vi "Unpack Goal Target Info.vi"(6 "Right Goal":T1, 8 "Left Goal":T1) -> (0 "Goal Found":bool, 1 "Target Y Angle (Cam relative)":dbl, 2 "Target X Angle (Cam relative)":dbl)   [LabVIEW 2013]
uses:
  Common Code/Goal Info.ctl
  Robot Global Data.vi
panel:
  # "CAMERA RELATIVE"
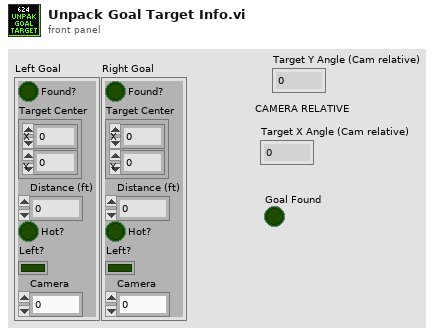
[diagram p1: front panel]
types:
  T1 = typedef "Goal Info.ctl" = cluster{"Found?":bool, "Target Center":cluster{"X":dbl, "Y":dbl}, "Distance (ft)":dbl, "Hot?":bool, "Left?":bool, "Camera":i16}
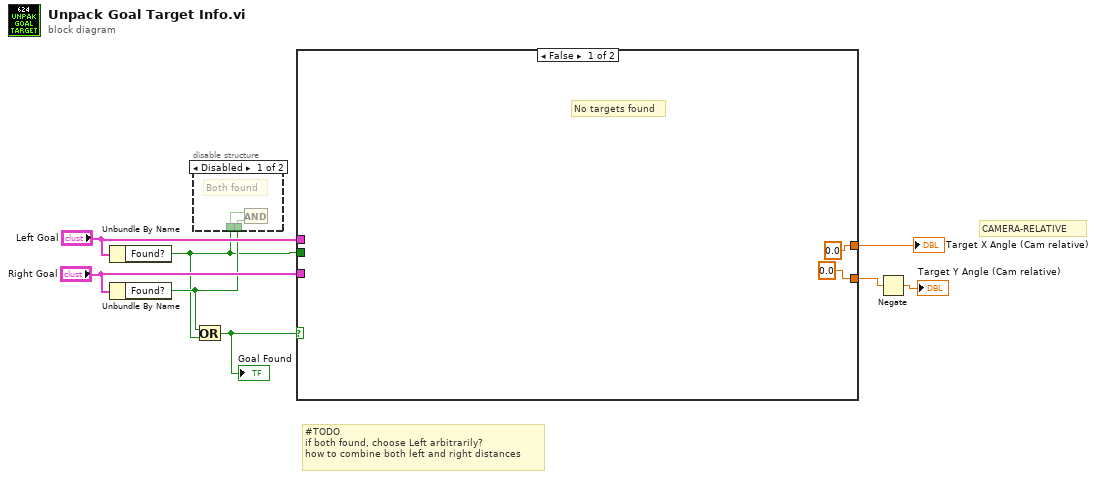
[diagram p0: block diagram]
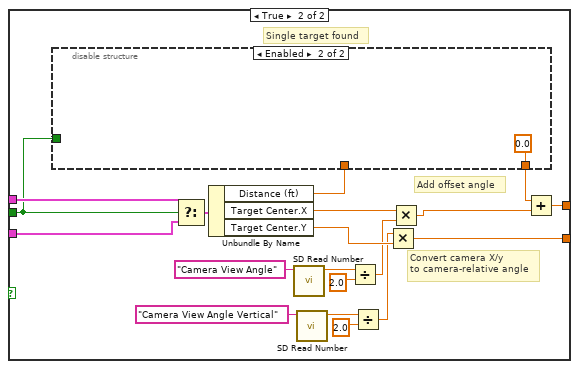
[diagram p2: hidden frame]
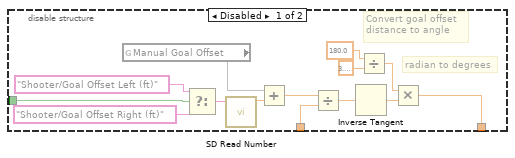
[diagram p3: hidden frame]
diagram:
  # "CAMERA-RELATIVE"
  # "#TODO\nif both found, choose Left arbitrarily?\nhow to combine both left and right distances"
  n1 = Unbundle By Name("Left Goal") -> ("Found?"=w4:bool)
  n2 = Unbundle By Name("Right Goal") -> ("Found?"=w5:bool)
  n3 = disable-structure shown="Disabled" {
    disable-tunnel: w5 -> [w10 _]
    disable-tunnel: w4 -> [w9 _]
    frame Disabled {
      # "Both found"
      n4 = And(x=w9, y=w10) -> ()  [unwired: 1 out]
    }
    frame Enabled {
    }
  }
  n5 = Or(x=w5, y=w4) -> (x .or. y?=w3:bool)
  "Goal Found" <- w3
  n6 = case shown="False" w3 {
    tunnel: "Left Goal" -> [_ w31]
    tunnel: "Right Goal" -> [_ w29]
    tunnel: [0.0 ("X") w27] -> w6
    tunnel: w4 -> [_ w28]
    tunnel: [0.0 ("X") w17] -> w1
    frame False {
      # "No targets found"
    }
    frame True {
      # "Convert camera X/y\nto camera-relative angle"
      # "Add offset angle"
      # "Single target found"
      n7 = Select(t=w31, s=w28, f=w29) -> (s? t:f=w30:T1)
      n8 = Unbundle By Name(w30) -> ("Distance (ft)"=w25:dbl, "Target Center.X"=w21:dbl, "Target Center.Y"=w19:dbl)
      n9 = disable-structure shown="Enabled" {
        disable-tunnel: w28 -> [w43 _]
        disable-tunnel: [w36 0.0] -> w26
        disable-tunnel: w25 -> [w35 _]
        frame Disabled {
          # "Convert goal offset\ndistance to angle"
          # "radian to degrees"
          n10 = global read "Robot Global Data.vi" "Manual Goal Offset"() -> (w32)
          n11 = Select(t="Shooter/Goal Offset Left (ft)" ("Name"), s=w43, f="Shooter/Goal Offset Right (ft)" ("Name")) -> (s? t:f=w42:string)
          n12 = call <vilib>:"SD Read Number.vi"("Name"=w42) -> ("Numeric"=w34:dbl)  [unwired: 8 in, 2 out]
          n13 = Add(x=w32, y=w34) -> (x+y=w33:dbl)
          n14 = Divide(x=w33, y=w35) -> (x/y=w41:dbl)
          n15 = Inverse Tangent(1:w41) -> (0:w40:dbl)
          n16 = Divide(x=180.0, y=3.141592653589793) -> (x/y=w39:dbl)
          n17 = Multiply(x=w39, y=w40) -> (x*y=w36:dbl)
        }
        frame Enabled {
        }
      }
      n18 = call <vilib>:"SD Read Number.vi"("Name"="Camera View Angle") -> ("Numeric"=w23:dbl)  [unwired: 8 in, 2 out]
      n19 = call <vilib>:"SD Read Number.vi"("Name"="Camera View Angle Vertical") -> ("Numeric"=w15:dbl)  [unwired: 8 in, 2 out]
      n20 = Divide(x=w23, y=2.0) -> (x/y=w18:dbl)
      n21 = Divide(x=w15, y=2.0) -> (x/y=w13:dbl)
      n22 = Multiply(x=w13, y=w19) -> (x*y=w17:dbl)
      n23 = Multiply(x=w21, y=w18) -> (x*y=w20:dbl)
      n24 = Add(x=w26, y=w20) -> (x+y=w27:dbl)
    }
  }
  "Target X Angle (Cam relative)" <- w6
  n25 = Negate(x=w1) -> (-x=→"Target Y Angle (Cam relative)":dbl)
